vi "SECoP-addProperty.vi"(8 "error in (no error)":errorcluster, 9 "property value (SECoP_data)":T1 {"ptr64" format="%.0x"; "ptr32" format="%.0x"}, 10 "property name":string, 11 "DLL path (in)":T2) -> (0 "error out":errorcluster, 3 "DLL path (out)":T2)   [LabVIEW 2023, in "SECoP.lvlib"]
doc: "Call <b>\"SECoP-addProperty.vi\"</b> to append a SECoP property to the last SEC node, module, command or parameter. You propably need this function or some of the convenience functions \"SECoP-addProperty*.vi\", because there are mandatory and some optional properties for everything.\n\n<b>DLL path</b> input and output of cluster from \"SECoP-Initialize.vi\"\n<b>property name</b> name of property\n<b>property value (SECoP_data)</b> value of the property"
uses:
  SECoP.lvlib
  SECoP-libraries.ctl
  SECoP-data/SECoP-data.ctl
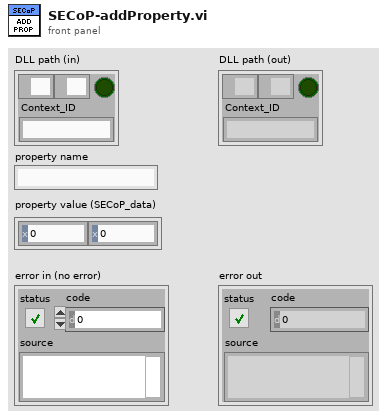
[diagram p1: front panel]
types:
  T1 = typedef "SECoP.lvlib/SECoP-data.ctl" = cluster{"ptr32":u32, "ptr64":u64}
  T2 = typedef "SECoP.lvlib/SECoP-libraries.ctl" = cluster{"serverDLL":path, "variantDLL":path, "cleanup_mode":bool, "Context_ID":string}
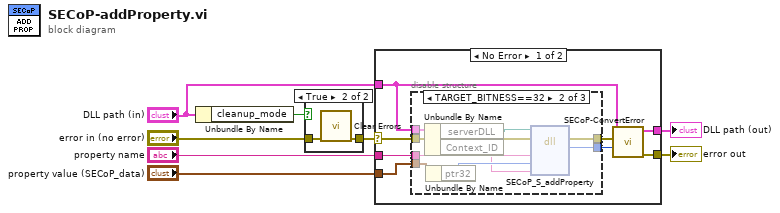
[diagram p0: block diagram]
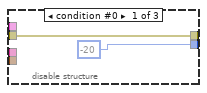
[diagram p3: hidden frame]
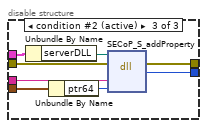
[diagram p4: hidden frame]
diagram:
  n1 = Unbundle By Name("DLL path (in)") -> ("cleanup_mode"=w5:bool)
  n2 = case shown="True" w5 {
    tunnel: "error in (no error)" -> [w9 w11]
    tunnel: [w9 w10] -> w3
    frame False {
    }
    frame True {
      n3 = call <vilib>:"Clear Errors.vi"("error in (no error)"=w11) -> ("error out"=w10:errorcluster)  [unwired: 5 in, 1 out]
    }
  }
  n4 = case shown="No Error" w3 {
    selector: w3 -> [w16 w39]
    tunnel: "DLL path (in)" -> [w12 w40]
    tunnel: [w18 w40] -> w8
    tunnel: [w19 w39] -> w7
    tunnel: "property name" -> [w15 _]
    tunnel: "property value (SECoP_data)" -> [w14 _]
    frame No Error {
      n5 = disable-structure shown="TARGET_BITNESS==32" {
        disable-tunnel: [w20 w30 w38] -> w17
        disable-tunnel: w16 -> [w20 w29 w37]
        disable-tunnel: w12 -> [_ w28 w36]
        disable-tunnel: w15 -> [_ w27 w35]
        disable-tunnel: w14 -> [_ w25 w33]
        disable-tunnel: [-20 w26 w34] -> w13
        frame condition #0 {
        }
        frame condition #1 {
          n6 = Unbundle By Name(w28) -> ("serverDLL"=w23:path, "Context_ID"=w22:string)
          n7 = Unbundle By Name(w25) -> ("ptr32"=w24:u32)
          n8 = dll-call lib="Z:/Praktische Aufgaben/SECoP-LabVIEW2015/32bit/SECoP32.dll" fn="SECoP_S_addProperty"(path in=w23, error in=w29, "Name"=w27, "Value"=w24, "szContextID"=w22) -> (error out=w30:errorcluster, "return type"=w26:i32)  [unwired: 4 in, 1 out]
        }
        frame condition #2 (active) {
          n9 = Unbundle By Name(w36) -> ("serverDLL"=w31:path)
          n10 = Unbundle By Name(w33) -> ("ptr64"=w32:u64)
          n11 = dll-call lib="Z:/Praktische Aufgaben/SECoP-LabVIEW2015/32bit/SECoP32.dll" fn="SECoP_S_addProperty"(path in=w31, error in=w37, "Name"=w35, "Value"=w32) -> (error out=w38:errorcluster, "return type"=w34:i32)  [unwired: 3 in, 1 out]
        }
      }
      n12 = call "SECoP-ConvertError.vi"("return code"=w13, "error in (no error)"=w17, "DLL path (in)"=w12) -> ("error out"=w19:errorcluster, "DLL path (out)"=w18:T2)  [unwired: 7 in]
    }
    frame Error {
    }
  }
  "DLL path (out)" <- w8
  "error out" <- w7
